vi "Manager.vi"(7 "Action":T1, 8 "Error In":errorcluster, 11 "Set Value":variant) -> (0 "Error Out":errorcluster)   [LabVIEW 2018, in "Toolkit.lvlib" / "File.lvlib"]
uses:
  File.lvlib
  Action.ctl
  Type Definitions/Statement.ctl
  Type Definitions/Tag.ctl
  Create ISO 8601 File Name.vi
  Write Header.vi
  Create Calendar Folder Tree.vi
  Get Oldest File.vi
  <vilib>/Utility/libraryn.llb/Check if File or Folder Exists.vi
  Create Bulk CSV String.vi
  Toolkit.lvlib
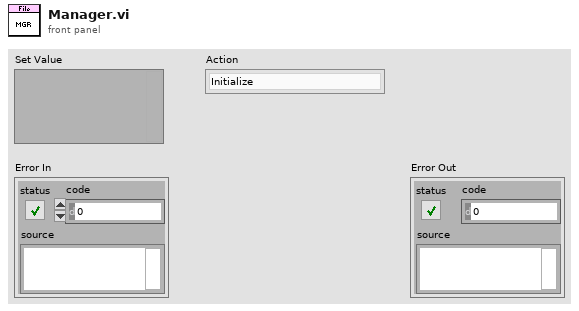
[diagram p1: front panel]
types:
  T1 = typedef "Toolkit.lvlib/File.lvlib/Action.ctl" = enum16{"Initialize", "Set Maximum File Size", "Set Maximum File Count", "Set Root Folder", "Set Enable Calendar Folder Tree", "Set File Extension", "Set Prune All", "Set Delimiter", "Start", "Write", "Stop", "Shutdown"}
  T2 = cluster{"Delete All Excessive":bool, "Delimiter":string, "Enable Calendar Tree":bool, "File Extension":string, "Time Stamp Format":string}
  T3 = typedef "Toolkit.lvlib/Statement.ctl" = cluster{"Time Stamp":timestamp, "Tag":T4, "Source":string, "Message":string}
  T4 = typedef "Toolkit.lvlib/Tag.ctl" = enum16{"Fatal", "Error", "Warn", "Info", "Debug", "Trace"}
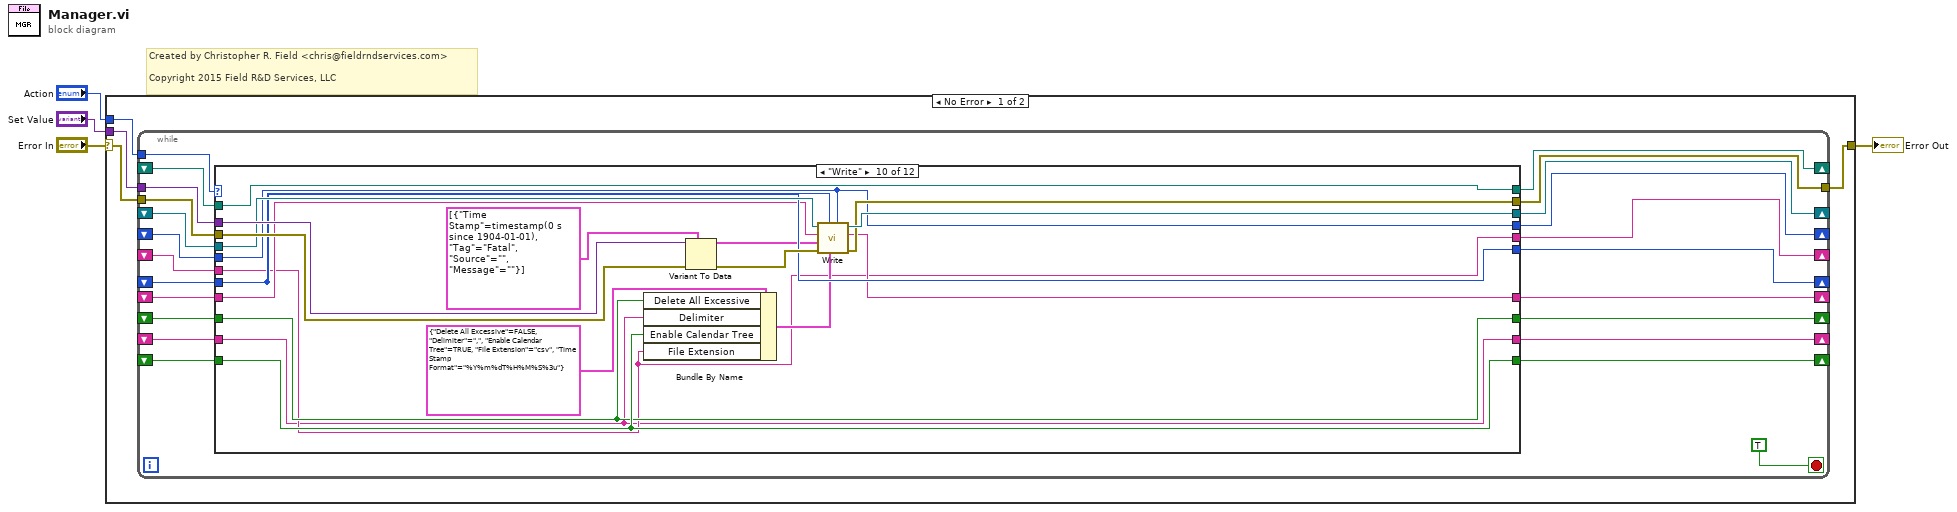
[diagram p0: block diagram]
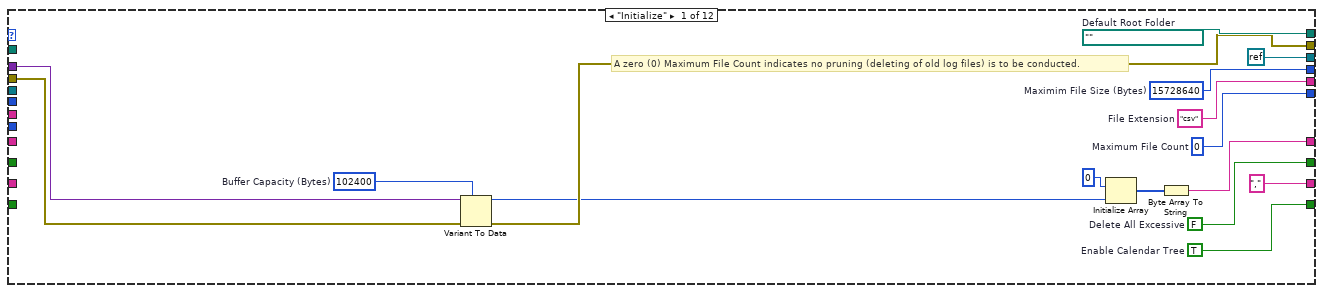
[diagram p2: hidden frame]
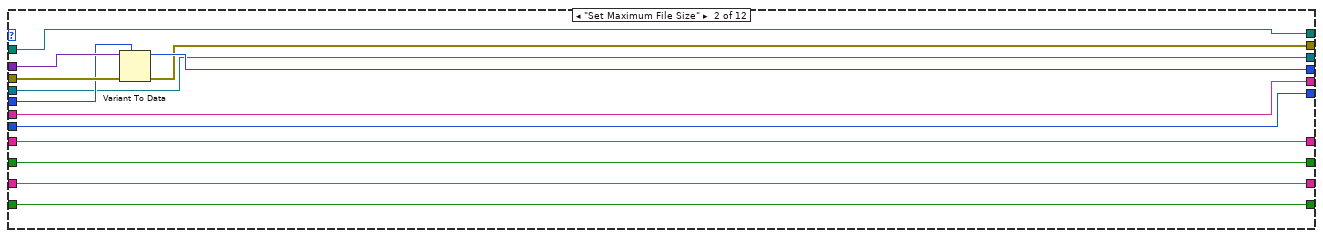
[diagram p3: hidden frame]
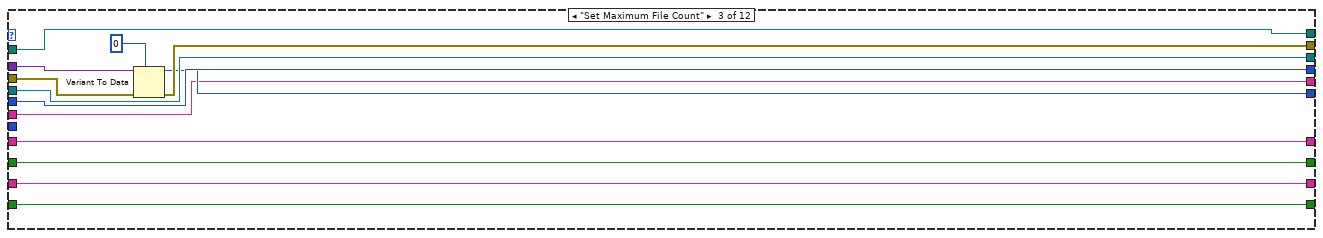
[diagram p4: hidden frame]
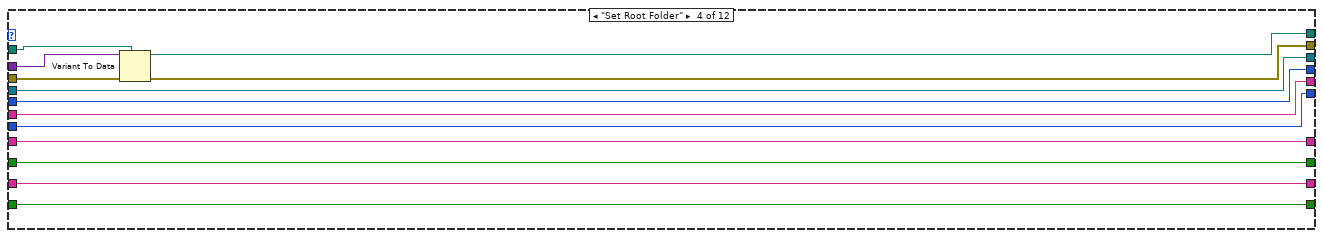
[diagram p5: hidden frame]
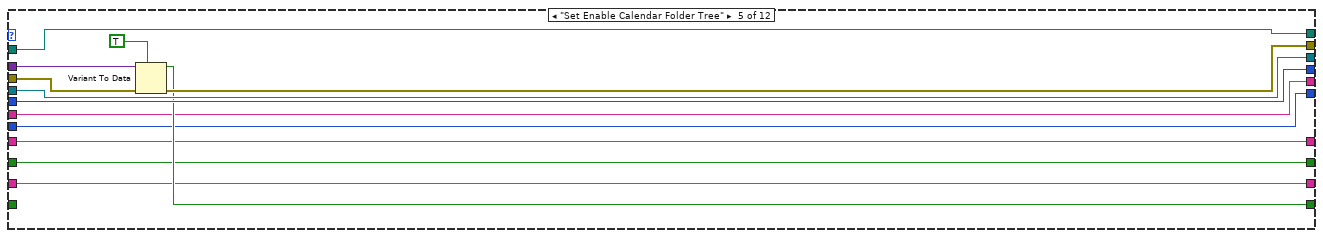
[diagram p6: hidden frame]
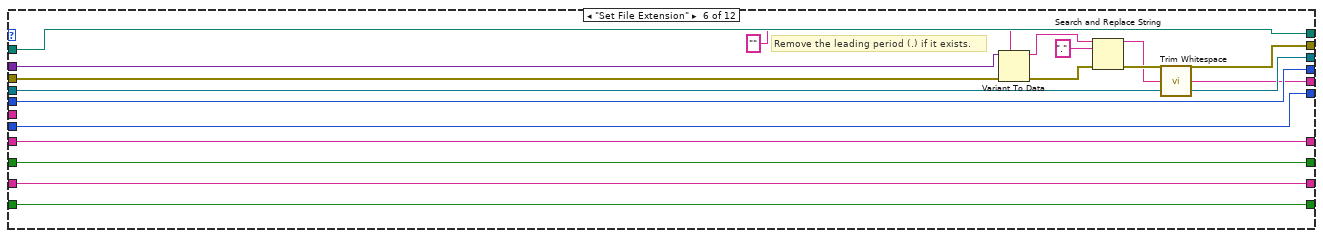
[diagram p7: hidden frame]
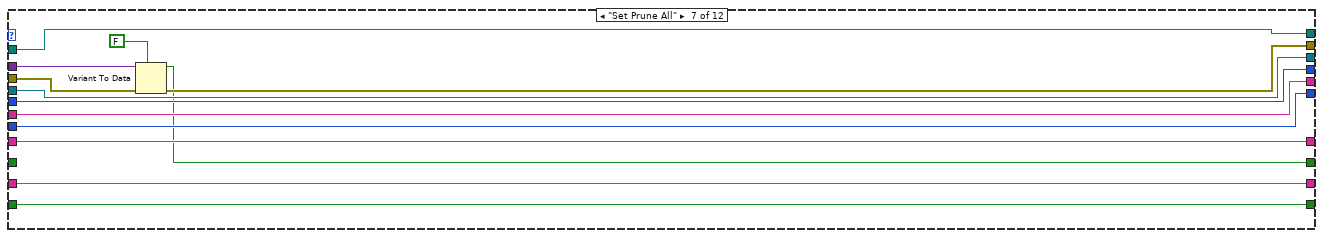
[diagram p8: hidden frame]
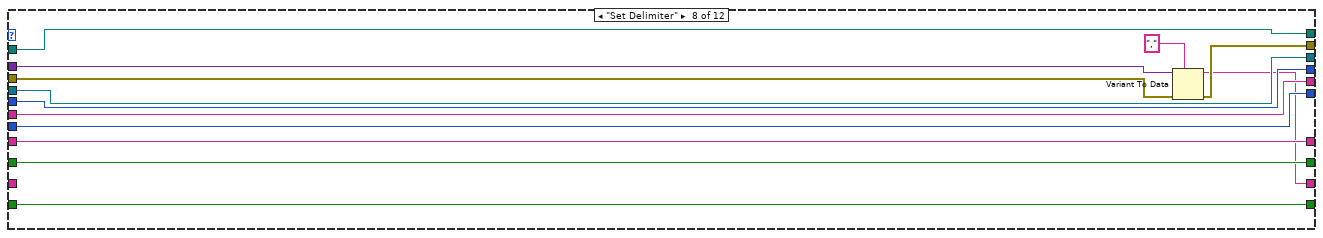
[diagram p9: hidden frame]
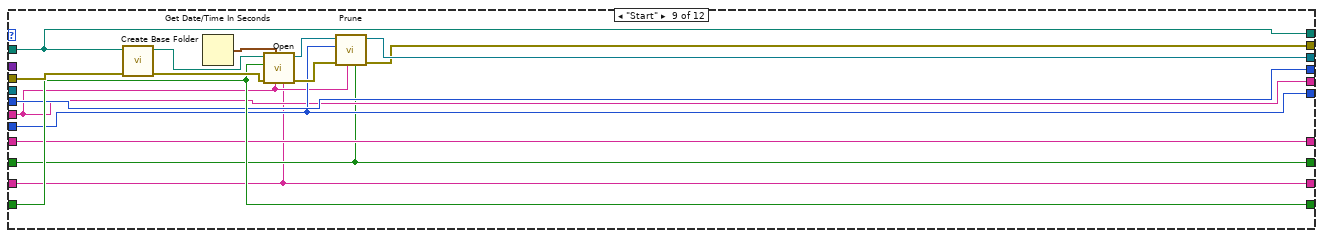
[diagram p10: hidden frame]
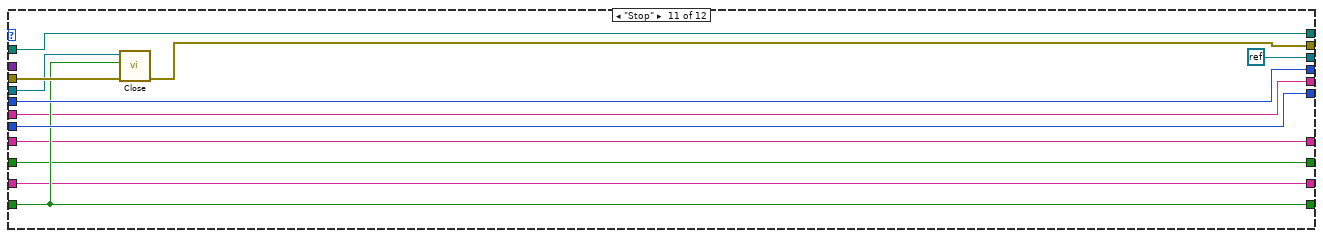
[diagram p11: hidden frame]
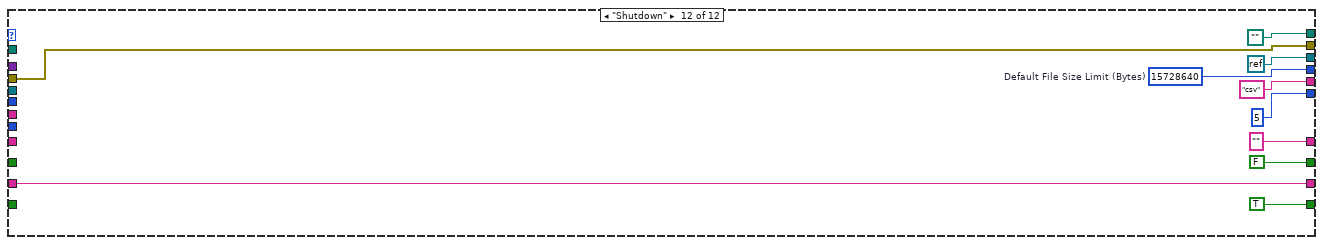
[diagram p12: hidden frame]
diagram:
  # "Created by Christopher R. Field <chris@fieldrndservices.com>\n\nCopyright 2015 Field R&D Services, LLC"
  n1 = case shown="No Error" "Error In" {
    selector: "Error In" -> [w7 w200]
    tunnel: "Action" -> [w8 _]
    tunnel: "Set Value" -> [w6 _]
    tunnel: [w5 w200] -> w1
    frame No Error {
      n2 = while {
        tunnel: w8 -> [w30]
        shift-right: [w29] -> _
        shift-left: _ -> [w24]
        shift-right: [w28] -> _
        shift-left: _ -> [w21]
        shift-right: [w27] -> _
        shift-left: _ -> [w22]
        tunnel: w7 -> [w26]
        tunnel: w6 -> [w25]
        tunnel: [w23] -> w5
        shift-right: [w20] -> _
        shift-left: _ -> [w19]
        shift-right: [w18] -> _
        shift-left: _ -> [w17]
        shift-right: [w16] -> _
        shift-left: _ -> [w15]
        shift-right: [w14] -> _
        shift-left: _ -> [w13]
        shift-right: [w12] -> _
        shift-left: _ -> [w11]
        shift-right: [w10] -> _
        shift-left: _ -> [w9]
        stop <- TRUE stop-if-true
        n3 = case shown="\"Write\"" w30 {
          tunnel: [w47 w57 w67 w86 w99 w116 w129 w142 w148 w169 w185 w196] -> w29
          tunnel: [refnum<k0> refnum w54 w69 w80 w95 w113 w126 w139 w151 w171 refnum<k0> refnum refnum<k0> refnum] -> w28
          tunnel: [w45 w55 w70 w82 w94 w112 w125 w138 w155 w174 w186 path ""] -> w27
          tunnel: w26 -> [w44 w60 w73 w84 w97 w114 w127 w140 w156 w176 w189 w198]
          tunnel: w25 -> [w39 w59 w72 w85 w98 w115 w128 w141 _ w177 _ _]
          tunnel: w24 -> [_ w58 w67 w86 w99 w116 w129 w142 w148 w169 w185 _]
          tunnel: [w40 w56 w71 w81 w96 w107 w120 w134 w149 w170 w184 w198] -> w23
          tunnel: w22 -> [_ w55 w70 w83 w94 w112 w125 w138 w155 w174 w186 _]
          tunnel: w21 -> [_ w54 w69 w80 w95 w113 w126 w139 _ w172 w188 _]
          tunnel: [w43 w53 w68 w79 w92 w109 w123 w136 w152 w162 w182 TRUE] -> w20
          tunnel: w19 -> [_ w53 w68 w79 _ w109 w123 w136 w152 w162 w182 _]
          tunnel: [w42 w52 w65 w78 w91 w111 w124 w137 w147 w168 w183 5] -> w18
          tunnel: w17 -> [_ w52 _ w78 w91 w111 w124 w137 w147 w168 w183 _]
          tunnel: [w41 w51 w64 w77 w90 w103 w119 w133 w145 w160 w181 "csv"] -> w16
          tunnel: w15 -> [_ w51 w64 w77 w90 _ w119 w133 w145 w160 w181 _]
          tunnel: [w34 w50 w63 w76 w89 w102 w122 w135 w146 w167 w180 "" ("Bulk CSV Buffer Out")] -> w14
          tunnel: w13 -> [_ w50 w63 w76 w89 w102 w122 w135 w146 w166 w180 _]
          tunnel: [w33 w49 w62 w75 w88 w101 w118 w132 w144 w161 w179 FALSE ("Delete All Excessive")] -> w12
          tunnel: w11 -> [_ w49 w62 w75 w88 w101 _ w132 w144 w161 w179 _]
          tunnel: ["," w48 w61 w74 w87 w100 w117 w130 w143 w159 w178 w190] -> w10
          tunnel: w9 -> [_ w48 w61 w74 w87 w100 w117 _ w143 w159 w178 w190]
          frame "Initialize" {
            w33 = FALSE  # Delete All Excessive
            w38 = 102400  # Buffer Capacity (Bytes)
            w41 = "csv"  # File Extension
            w42 = 0  # Maximum File Count
            w43 = TRUE  # Enable Calendar Tree
            w45 = path ""  # Default Root Folder
            w47 = i64 15728640  # Maximim File Size (Bytes)
            # "A zero (0) Maximum File Count indicates no pruning (deleting of old log files) is to be conducted."
            n4 = Variant To Data(error in=w44, type=w38, Variant=w39) -> (data=w37:i32, error out=w40:errorcluster)
            n5 = Initialize Array(u8 0, w37) -> (w35:u8[])
            n6 = Byte Array To String(unsigned byte array=w35) -> (string=w34:string)
          }
          frame "Set Maximum File Size" {
            n7 = Variant To Data(error in=w60, type=w58, Variant=w59) -> (data=w57:i64, error out=w56:errorcluster)
          }
          frame "Set Maximum File Count" {
            n8 = Variant To Data(error in=w73, type=0, Variant=w72) -> (data=w65:i32, error out=w71:errorcluster)
          }
          frame "Set Root Folder" {
            n9 = Variant To Data(error in=w84, type=w83, Variant=w85) -> (data=w82:path, error out=w81:errorcluster)
          }
          frame "Set Enable Calendar Folder Tree" {
            n10 = Variant To Data(error in=w97, type=TRUE, Variant=w98) -> (data=w92:bool, error out=w96:errorcluster)
          }
          frame "Set File Extension" {
            # "Remove the leading period (.) if it exists."
            n11 = Variant To Data(error in=w114, type="", Variant=w115) -> (data=w106:string, error out=w108:errorcluster)
            n12 = Search and Replace String(input string=w106, search string=".", error in=w108) -> (result string=w104:string, error out=w107:errorcluster)  [unwired: 5 in, 2 out]
            n13 = call <vilib>:"Trim Whitespace.vi"("string"=w104) -> ("trimmed string"=w103:string)  [unwired: 1 in]
          }
          frame "Set Prune All" {
            n14 = Variant To Data(error in=w127, type=FALSE, Variant=w128) -> (data=w118:bool, error out=w120:errorcluster)
          }
          frame "Set Delimiter" {
            n15 = Variant To Data(error in=w140, type=",", Variant=w141) -> (data=w130:string, error out=w134:errorcluster)
          }
          frame "Start" {
            n16 = call "Create Base Folder.vi"("Error In"=w156, "Root Folder"=w155) -> ("Error Out"=w157:errorcluster, "Base Folder"=w158:path)  [unwired: 8 in]
            n17 = Get Date/Time In Seconds() -> (seconds since 1Jan1904=w153:timestamp)
            n18 = call "Open.vi"("Delimiter"=w143, "File Extension"=w145, "Start Time Stamp"=w153, "Error In"=w157, "Enable Calendar Tree"=w152, "Base Folder"=w158) -> ("Error Out"=w150:errorcluster, "Log Out"=w154:refnum<file>)  [unwired: 4 in]
            n19 = call "Prune.vi"("Delete All Excessive"=w144, "File Extension"=w145, "Error In"=w150, "Maximum File Count"=w147, "File In"=w154) -> ("Error Out"=w149:errorcluster, "File Out"=w151:refnum<file>)  [unwired: 5 in]
          }
          frame "Write" {
            n20 = Bundle By Name(cluster=T2 {"Delete All Excessive"=FALSE, "Delimiter"=",", "Enable Calendar Tree"=TRUE, "File Extension"="csv", "Time Stamp Format"="%Y%m%dT%H%M%S%3u"} ("Options"), "Delete All Excessive"=w161, "Delimiter"=w159, "Enable Calendar Tree"=w162, "File Extension"=w160) -> (w163:T2)
            n21 = Variant To Data(error in=w176, type=T3[] [{"Time Stamp"=timestamp(0 s since 1904-01-01), "Tag"=enum."Fatal", "Source"="", "Message"=""}], Variant=w177) -> (data=w165:T3[], error out=w173:errorcluster)
            n22 = call "Write.vi"("Maximum File Size (Bytes)"=w169, "Options"=w163, "Maximum File Count"=w168, "Error In"=w173, "Messages"=w165, "Bulk CSV Buffer In"=w166, "Log In"=w172) -> ("Error Out"=w170:errorcluster, "Bulk CSV Buffer Out"=w167:string, "Log Out"=w171:refnum<file>)  [unwired: 2 in]
          }
          frame "Stop" {
            n23 = call "Close.vi"("Error In"=w189, "Enable Calendar Tree"=w182, "Log In"=w188) -> ("Error Out"=w184:errorcluster)  [unwired: 7 in, 1 out]
          }
          frame "Shutdown" {
            w196 = i64 15728640  # Default File Size Limit (Bytes)
          }
        }
      }
    }
    frame Error {
    }
  }
  "Error Out" <- w1
